vi "Teleop.vi"(9 "navX Device \nTypeDef":T1={"Interface"={"Protocol"=enum."SPI", "Update Rate (4Hz-60Hz)"=50, "navX Open TypeDef"=variant(cluster{"DevStatus":errorcluster, "Handle":i32, "Controller":enum16{"Controller 1"}, "SPI Bus":enum16{"SPI On-Board, CS0", "SPI On-Board, CS1", "SPI On-Board, CS2", "SPI On-Board, CS3", "SPI MXP", "Invalid"}} {"DevStatus"={"status"=FALSE, "code"=0, "source"=""}, "Handle"=0, "Controller"=enum."Controller 1", "SPI Bus"=enum."SPI On-Board, CS0"})}, "Notify Packet"=refnum, "Loop VI Refnum"=refnum, "Ready to Close Occurrence Refnum"=refnum} {"Interface"."Update Rate (4Hz-60Hz)" min=4 max=60 step=1}, 10 "Match Info":T3={"Autonomous Elapsed Seconds"=0.0, "TeleOp Elapsed Seconds"=0.0, "Disabled Elapsed Seconds"=0.0, "Visited Autonomous"=FALSE, "Visited TeleOp"=FALSE, "Visited Disabled"=FALSE, "Autonomous Settings"={"Autonomous Style"=enum."Independent", "VI Refnum"=refnum}}, 11 "Call Context":T4) -> ()   [LabVIEW 2014]
doc: "This VI is called for each TeleOp packet received from the DS where the robot is not disabled. It is often used to read from the joysticks and update I/O or to update setpoints for timed control loops. It should complete and return within 20 milliseconds or it may miss DS packets."
uses:
  <vilib>/Rock Robotics/WPI/DriverStation/WPI_DriverStationDerivedRobotMode.ctl
  <vilib>/Rock Robotics/WPI/DriverStation/WPI_DriverStationMatch Info.ctl
  navX Library v2/TypeDefs/Z900_navX_DeviceTypeDef.ctl
  navX Library v2/TypeDefs/Z900_navX_ProtocolTypeDef.ctl
  navX Library v2/TypeDefs/Z900_navX_NotifyPacketTypeDef.ctl
  navX Library v2/TypeDefs/Z900_navX_ActionTypeDef.ctl
  <vilib>/Rock Robotics/WPI/Joystick/WPI_JoystickGetSetRefNum.vi
  <vilib>/Rock Robotics/Network Tables/SD Write Boolean Array.vi
  <vilib>/Rock Robotics/Network Tables/SD Write Numeric Array.vi
  <vilib>/Rock Robotics/Network Tables/SD Read Boolean.vi
  <vilib>/Rock Robotics/Network Tables/SD Read Number.vi
  <vilib>/Rock Robotics/WPI/RobotDrive/WPI_RobotDriveGetSetRefNum.vi
  <vilib>/Rock Robotics/WPI/RobotDrive/WPI_RobotDriveMecanumDrive_Cartesian.vi
  navX Library v2/navX Library v2.lvlib
panel:
  out "Sample Slider 0":dbl(slide) scale=0.0..5.0
  out "Sample Boolean 1":bool
  out "Sample Boolean 0":bool
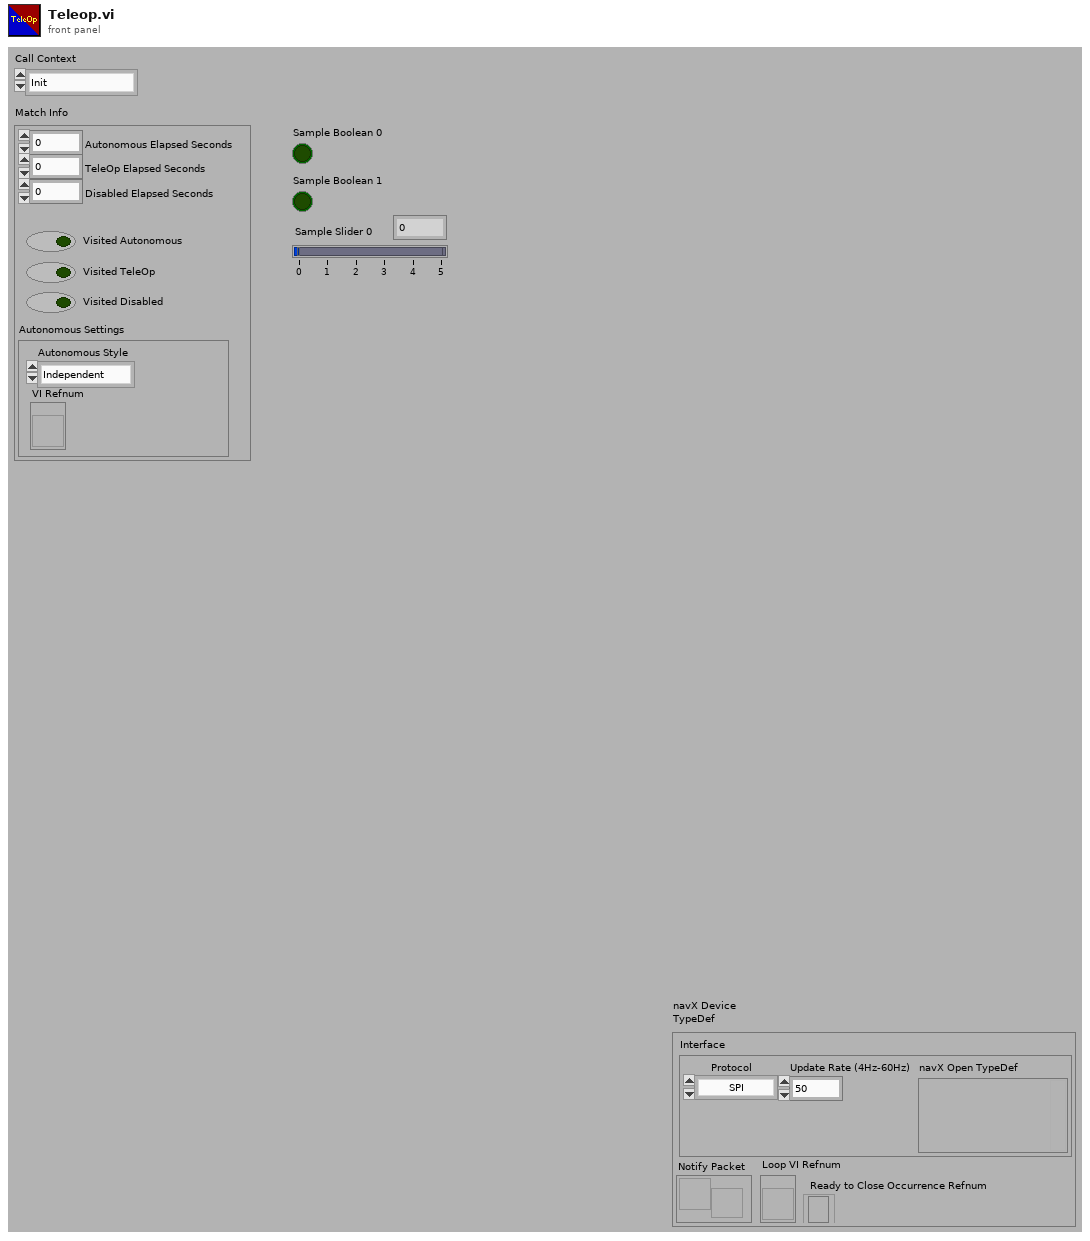
[diagram p1: front panel]
types:
  T1 = typedef "navX Library v2.lvlib/Z900_navX_DeviceTypeDef.ctl" = cluster{"Interface":cluster{"Protocol":T2, "Update Rate (4Hz-60Hz)":u8, "navX Open TypeDef":variant}, "Notify Packet":refnum<notifier>, "Loop VI Refnum":refnum<vi>, "Ready to Close Occurrence Refnum":refnum<k4>}
  T2 = typedef "navX Library v2.lvlib/Z900_navX_ProtocolTypeDef.ctl" = enum16{"SERIAL", "I2C", "SPI"}
  T3 = typedef "WPI_DriverStationMatch Info.ctl" = cluster{"Autonomous Elapsed Seconds":dbl, "TeleOp Elapsed Seconds":dbl, "Disabled Elapsed Seconds":dbl, "Visited Autonomous":bool, "Visited TeleOp":bool, "Visited Disabled":bool, "Autonomous Settings":cluster{"Autonomous Style":enum16{"Iterative", "Independent"}, "VI Refnum":refnum<vi>}}
  T4 = typedef "WPI_DriverStationDerivedRobotMode.ctl" = enum16{"Init", "Execute", "Stop"}
  T5 = typedef "WPI_RobotDriveDevRef.ctl" = cluster{"DevStatus":errorcluster, "Motors[]":T6[], "Square Inputs":bool, "Max Output":dbl}
  T6 = typedef "WPI_MotorControlDeviceRef.ctl" = cluster{"DeviceStatus":errorcluster, "Type":T7, "PWM":cluster{"Controller":T8, "PWM Channel":T9, "DeadBand":T10}, "CAN":cluster{"Device Number":u8, "Control Mode":T11, "Semaphore":T12, "Max Vout":dbl, "TalonSRX Control Mode":T13}, "Invert":bool, "TransformRef":T14, "InvTransformRef":T14}
  T7 = typedef "WPI_MotorControlType.ctl" = enum16{"PWM", "CAN", "CANTalonSRX"}
  T8 = typedef "FPGA_TypedefDigitalModule.ctl" = enum16{"Controller 1"}
  T9 = typedef "FPGA_DIOPWMChannel.ctl" = enum8{"PWM 0", "PWM 1", "PWM 2", "PWM 3", "PWM 4", "PWM 5", "PWM 6", "PWM 7", "PWM 8", "PWM 9", "PWM MXP 0", "PWM MXP 1", "PWM MXP 2", "PWM MXP 3", "PWM MXP 4", "PWM MXP 5", "PWM MXP 6", "PWM MXP 7", "PWM MXP 8", "PWM MXP 9", "Invalid"}
  T10 = typedef "WPI_PWMDeadband.ctl" = cluster{"Name":string, "maxPositivePwm":i32, "minPositivePwm":i32, "centerPwm":i32, "maxNegativePwm":i32, "minNegativePwm":i32, "angularRange":u16}
  T11 = typedef "WPI_CANJaguar_ControlMode.ctl" = enum8{"Percent VBus", "Current", "Speed", "Position", "Voltage"}
  T12 = typedef "Semaphore RefNum" = refnum<k1>
  T13 = typedef "WPI_CANTalonSRX_APIControlMode.ctl" = enum8{"Percent VBus", "Speed", "Position", "Slave", "Unchanged / Invalid"}
  T14 = typedef "WPI_PWMTransform_ConPane.ctl" = refnum<vi>
  T15 = typedef "WPI_JoystickDevRef.ctl" = cluster{"Device":T16}
  T16 = typedef "WPI_JoystickDeviceEnum.ctl" = enum16{"USB 0", "USB 1", "USB 2", "USB 3", "USB 4", "USB 5"}
  T17 = cluster{"Yaw":dbl, "Roll":dbl, "Pitch":dbl, "Heading":dbl, "Fused Heading":dbl}
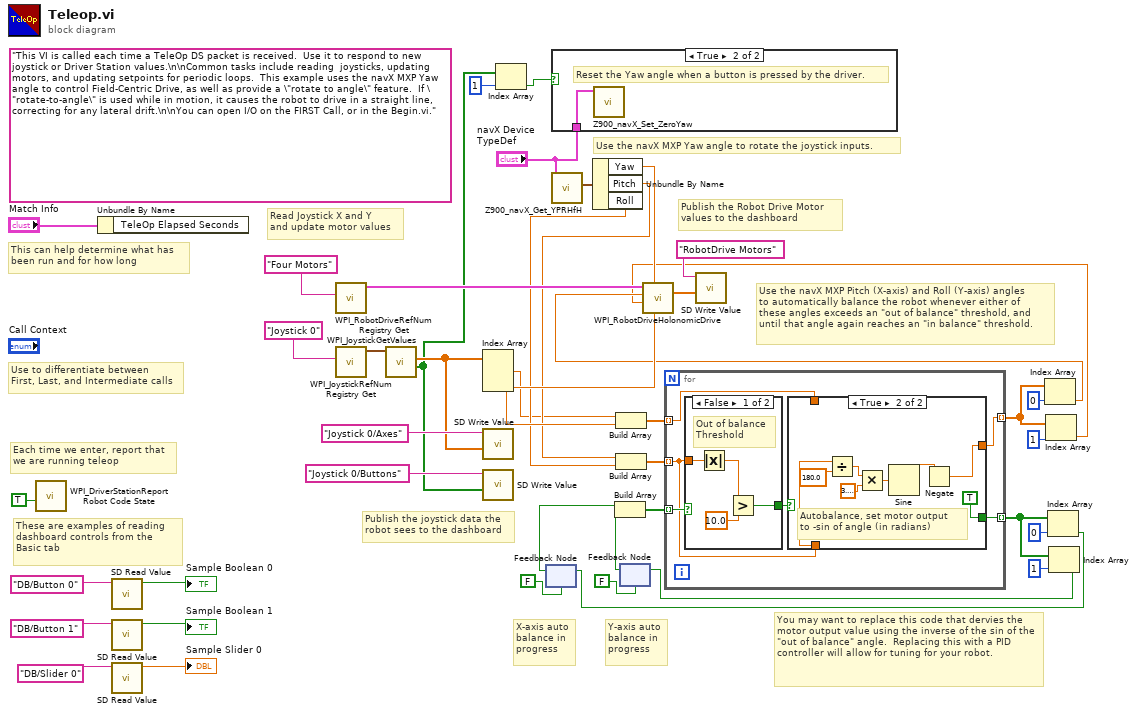
[diagram p0: block diagram]
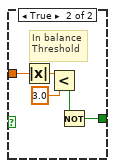
[diagram p3: hidden frame]
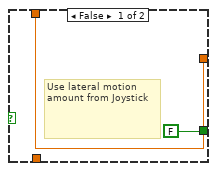
[diagram p4: hidden frame]
diagram:
  (unwired) "This VI is called each time a TeleOp DS packet is received.  Use it to respond to new joystick or Driver Station values.\n\nCommon tasks include reading  joysticks, updating motors, and updating setpoints for periodic loops.  This example uses the navX MXP Yaw angle to control Field-Centric Drive, as well as provide a \"rotate to angle\" feature.  If \"rotate-to-angle\" is used while in motion, it causes the robot to drive in a straight line, correcting for any lateral drift.\n\nYou can open I/O on the FIRST Call, or in the Begin.vi."
  # "You may want to replace this code that dervies the motor output value using the inverse of the sin of the \"out of balance\" angle.  Replacing this with a PID controller will allow for tuning for your robot."
  # "Y-axis auto\nbalance in \nprogress"
  # "X-axis auto\nbalance in \nprogress"
  # "Use the navX MXP Pitch (X-axis) and Roll (Y-axis) angles\nto automatically balance the robot whenever either of \nthese angles exceeds an \"out of balance\" threshold, and\nuntil that angle again reaches an \"in balance\" threshold."
  # "Use the navX MXP Yaw angle to rotate the joystick inputs."
  # "These are examples of reading dashboard controls from the Basic tab"
  # "Publish the Robot Drive Motor\nvalues to the dashboard"
  # "Publish the joystick data the\nrobot sees to the dashboard"
  # "Each time we enter, report that\nwe are running teleop"
  # "Use to differentiate between\nFirst, Last, and Intermediate calls"
  # "This can help determine what has\nbeen run and for how long"
  # "Read Joystick X and Y \nand update motor values"
  n1 = call <vilib>:"WPI_DriverStationReport Robot Code State.vi"("TeleOp"=TRUE ("Autonomous")) -> ()  [unwired: 10 in, 1 out]
  n2 = Unbundle By Name("Match Info") -> ()  [unwired: 1 out]
  n3 = call-poly <vilib>:"SD Read Value.vi"("Name"="DB/Button 0" ("refnum name")) -> ("Boolean"=→"Sample Boolean 0":bool)  [unwired: 8 in, 2 out]
  n4 = call-poly <vilib>:"SD Read Value.vi"("Name"="DB/Button 1" ("refnum name")) -> ("Boolean"=→"Sample Boolean 1":bool)  [unwired: 8 in, 2 out]
  n5 = call-poly <vilib>:"SD Read Value.vi"("Name"="DB/Slider 0" ("refnum name")) -> ("Numeric"=→"Sample Slider 0":dbl)  [unwired: 8 in, 2 out]
  n6 = call <vilib>:"WPI_RobotDriveRefNum Registry Get.vi"("refnum name"="Four Motors") -> ("RobotDriveDevRef"=w43:T5)  [unwired: 1 in, 9 out]
  n7 = call <vilib>:"WPI_JoystickRefNum Registry Get.vi"("refnum name"="Joystick 0") -> ("JoystickDevRef"=w41:T15)  [unwired: 1 in, 9 out]
  n8 = call <vilib>:"WPI_JoystickGetValues.vi"("JoystickDevRef"=w41) -> ("Buttons"=w24:bool[], "Axes"=w29:dbl[])  [unwired: 6 in, 3 out]
  n9 = Index Array(array=w29) -> (element #1=w2:dbl, element #2=w6:dbl, element #3=w23:dbl)  [unwired: 3 in]
  n10 = call-poly <vilib>:"SD Write Value.vi"("Numeric Array"=w29, "Name"="Joystick 0/Axes") -> ()  [unwired: 8 in, 2 out]
  n11 = call-poly <vilib>:"SD Write Value.vi"("Boolean Array"=w24, "Name"="Joystick 0/Buttons") -> ()  [unwired: 8 in, 2 out]
  n12 = Index Array(array=w24, index=1) -> (element=w1:bool)
  n13 = feedback #1(FALSE) -> (w20:bool)
  n14 = case shown="True" w1 {
    tunnel: "navX Device \nTypeDef" -> [_ w46]
    frame False {
    }
    frame True {
      # "Reset the Yaw angle when a button is pressed by the driver."
      n15 = call "Z900_navX_Set_ZeroYaw.vi"("navX Device"=w46) -> ()  [unwired: 9 in, 2 out]
    }
  }
  n16 = call "Z900_navX_Get_YPRHfH.vi"("navX Device"="navX Device \nTypeDef") -> ("YRPHfH"=w28:T17)  [unwired: 7 in, 3 out]
  n17 = Unbundle By Name(w28) -> ("Yaw"=w25:dbl, "Pitch"=w5:dbl, "Roll"=w4:dbl)
  n18 = Build Array(w2, w6) -> (w17:dbl[])
  n19 = Build Array(w5, w4) -> (w3:dbl[])
  n20 = feedback #2(FALSE) -> (w19:bool)
  n21 = Build Array(w20, w19) -> (w18:bool[])
  n22 = for {
    tunnel: w18 -> [w51] mode=indexing
    tunnel: w17 -> [w47] mode=indexing
    tunnel: [w50] -> w16 mode=indexing
    tunnel: [w49] -> w9 mode=indexing
    tunnel: w3 -> [w48] mode=indexing
    n23 = case shown="False" w51 {
      tunnel: w48 -> [w56 w59]
      tunnel: [w53 w58] -> w52
      frame False {
        # "Out of balance\nThreshold"
        n24 = Absolute Value(x=w56) -> (abs(x)=w55:dbl)
        n25 = Greater?(x=w55, y=10.0) -> (0:w53:bool)
      }
      frame True {
        # "In balance\nThreshold"
        n26 = Absolute Value(x=w59) -> (abs(x)=w60:dbl)
        n27 = Less?(x=w60, y=3.0) -> (x < y?=w57:bool)
        n28 = Not(x=w57) -> (.not. x?=w58:bool)
      }
    }
    n29 = case shown="True" w52 {
      tunnel: w48 -> [_ w70]
      tunnel: [w62 w64] -> w49
      tunnel: [FALSE TRUE] -> w50
      tunnel: w47 -> [w62 _]
      frame False {
        # "Use lateral motion amount from Joystick"
      }
      frame True {
        # "Autobalance, set motor output \nto -sin of angle (in radians)"
        n30 = Divide(x=w70, y=180.0) -> (x/y=w68:dbl)
        n31 = Multiply(x=w68, y=3.141592653589793) -> (x*y=w66:dbl)
        n32 = Sine(x=w66) -> (sin(x)=w65:dbl)
        n33 = Negate(x=w65) -> (-x=w64:dbl)
      }
    }
  }
  n34 = Index Array(array=w9, index=0) -> (element=w8:dbl)
  n35 = Index Array(array=w9, index=1) -> (element=w7:dbl)
  n36 = call-poly <vilib>:"WPI_RobotDriveHolonomicDrive.vi"("Rotation"=w23, "Gyro Angle"=w25, "Y"=w7, "X"=w8, "RobotDriveDevRef"=w43) -> ("Motor Values"=w30:dbl[])  [unwired: 4 in, 2 out]
  n37 = call-poly <vilib>:"SD Write Value.vi"("Numeric Array"=w30, "Name"="RobotDrive Motors") -> ()  [unwired: 8 in, 2 out]
  n38 = Index Array(array=w16, index=0) -> (element=w13:bool)
  n39 = feedback-in #1(w13) -> ()
  n40 = Index Array(array=w16, index=1) -> (element=w12:bool)
  n41 = feedback-in #2(w12) -> ()
